vi "Throber Control__jki_lib_user_interface -- VI Tester.vi"(6 "animate?":bool, 10 "static throber reference":refnum<vi>, 11 "animate throber reference":refnum<vi>) -> ()   [LabVIEW 2011]
uses:
  Throber List Animated__jki_lib_user_interface - VI Tester.ctl
panel:
  # "Copyright © 2006 James Kring, Inc. All rights reserved.\nMichael Aivaliotis michael.aivaliotis@jameskring.com\nalternate email: michael@aivaliotis.com\n\nThis library is provided \"AS IS\" , WITHOUT WARRANTIES OR \nCONDITIONS OF ANY KIND, either express or implied.\n\nJames Kring, Inc. -- http://www.jameskring.com"
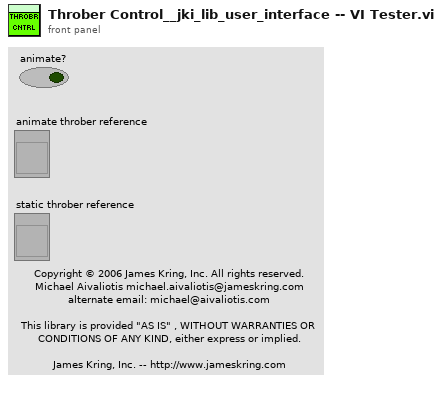
[diagram p1: front panel]
types:
  T1 = typedef "Throber List Animated__jki_lib_user_interface - VI Tester.ctl" = u16
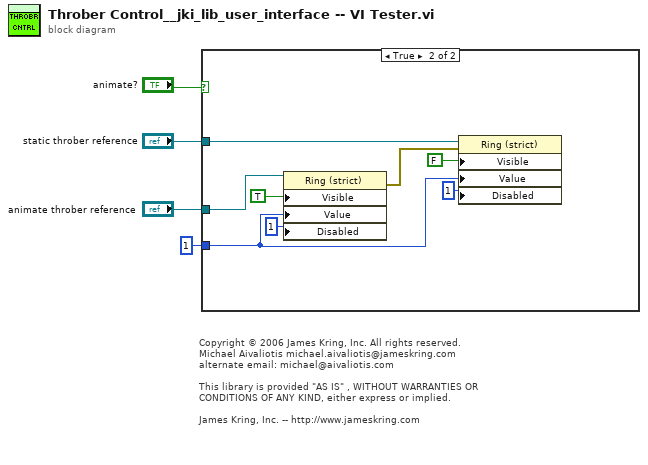
[diagram p0: block diagram]
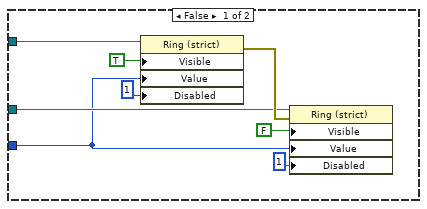
[diagram p2: hidden frame]
diagram:
  # "Copyright © 2006 James Kring, Inc. All rights reserved.\nMichael Aivaliotis michael.aivaliotis@jameskring.com\nalternate email: michael@aivaliotis.com\n\nThis library is provided \"AS IS\" , WITHOUT WARRANTIES OR \nCONDITIONS OF ANY KIND, either express or implied.\n\nJames Kring, Inc. -- http://www.jameskring.com"
  n1 = case shown="True" "animate?" {
    tunnel: "static throber reference" -> [w9 w20]
    tunnel: "animate throber reference" -> [w8 w18]
    tunnel: T1 1 ("Throber List") -> [w5 w13]
    frame False {
      n2 = property class="Ring (strict)"(reference=w9, "Visible"=TRUE, "Value"=w5, "Disabled"=u8 1) -> (error out=w10:errorcluster)  [unwired: 1 in, 1 out]
      n3 = property class="Ring (strict)"(reference=w8, error in=w10, "Visible"=FALSE, "Value"=w5, "Disabled"=u8 1) -> ()  [unwired: 2 out]
    }
    frame True {
      n4 = property class="Ring (strict)"(reference=w18, "Visible"=TRUE, "Value"=w13, "Disabled"=u8 1) -> (error out=w16:errorcluster)  [unwired: 1 in, 1 out]
      n5 = property class="Ring (strict)"(reference=w20, error in=w16, "Visible"=FALSE, "Value"=w13, "Disabled"=u8 1) -> ()  [unwired: 2 out]
    }
  }
